vi "LEP_RV_MemoryMap_SectionNames.vi"() -> (0 "Linker Names":string[](array[string]), 1 "All Section Names":string[](array[string]))   [LabVIEW 2011]
doc: "Return names for all section types."
uses:
  LEP_RV_MemoryMap_Sections.ctl
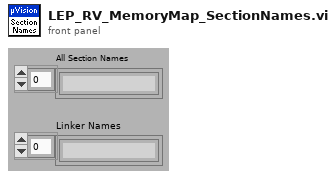
[diagram p1: front panel]
types:
  T1 = typedef "LEP_RV_MemoryMap_Sections.ctl" = enum16{"ROM1 (0)", "ROM2 (1)", "ROM3 (2)", "IROM1 (3)", "IROM2 (4)", "RAM1 (5)", "RAM2 (6)", "RAM3 (7)", "IRAM1 (8)", "IRAM2 (9)"}
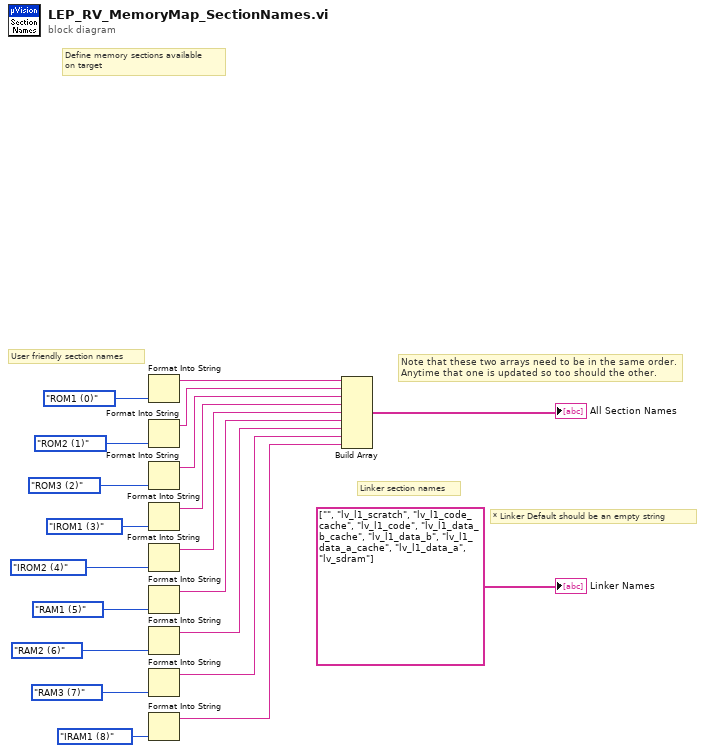
[diagram p0: block diagram]
diagram:
  # "* Linker Default should be an empty string"
  # "User friendly section names"
  # "Linker section names"
  # "Note that these two arrays need to be in the same order. \nAnytime that one is updated so too should the other."
  # "Define memory sections available\non target"
  n1 = Format Into String(LEP_RV_MemoryMap_Sections."ROM1 (0)" ("Section Type")) -> (resulting string=w18:string)  [unwired: 3 in, 1 out]
  n2 = Format Into String(LEP_RV_MemoryMap_Sections."ROM2 (1)" ("Section Type")) -> (resulting string=w1:string)  [unwired: 3 in, 1 out]
  n3 = Format Into String(LEP_RV_MemoryMap_Sections."ROM3 (2)" ("Section Type")) -> (resulting string=w10:string)  [unwired: 3 in, 1 out]
  n4 = Format Into String(LEP_RV_MemoryMap_Sections."IROM1 (3)" ("Section Type")) -> (resulting string=w9:string)  [unwired: 3 in, 1 out]
  n5 = Format Into String(LEP_RV_MemoryMap_Sections."IROM2 (4)" ("Section Type")) -> (resulting string=w8:string)  [unwired: 3 in, 1 out]
  n6 = Format Into String(LEP_RV_MemoryMap_Sections."RAM1 (5)" ("Section Type")) -> (resulting string=w7:string)  [unwired: 3 in, 1 out]
  n7 = Format Into String(LEP_RV_MemoryMap_Sections."RAM2 (6)" ("Section Type")) -> (resulting string=w6:string)  [unwired: 3 in, 1 out]
  n8 = Format Into String(LEP_RV_MemoryMap_Sections."RAM3 (7)" ("Section Type")) -> (resulting string=w5:string)  [unwired: 3 in, 1 out]
  n9 = Format Into String(LEP_RV_MemoryMap_Sections."IRAM1 (8)" ("Section Type")) -> (resulting string=w4:string)  [unwired: 3 in, 1 out]
  n10 = Build Array(w18, w1, w10, w9, w8, w7, w6, w5, w4) -> (→"All Section Names":string[])
  "Linker Names" <- string[] ["", "lv_l1_scratch", "lv_l1_code_cache", "lv_l1_code", "lv_l1_data_b_cache", "lv_l1_data_b", "lv_l1_data_a_cache", "lv_l1_data_a", "lv_sdram"]
